vi "ReleaseQueue.vi"   [LabVIEW 2013]
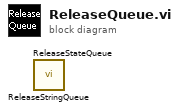
[diagram p0: block diagram]
diagram:
  n1 = call "ReleaseStringQueue.vi"() -> ()  [unwired: 11 in, 1 out]
  n2 = call "ReleaseStateQueue.vi"() -> ()  [unwired: 11 in, 1 out]
